vi "read_mote.vi"() -> (0 "DataSocket error":errorcluster, 1 "SF error":errorcluster)   [LabVIEW 2011]
panel:
  out "Sent Data":string
  out "Parsed Data":T1
  out "# Sent Data":u64
  out "Received data from mote":string
  out "Deque error":errorcluster
  # "DO NOT USE id 0 for a mote !"
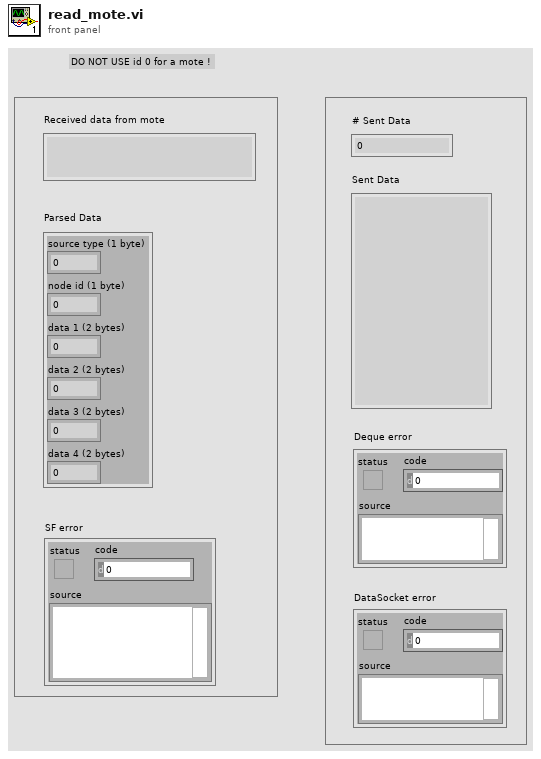
[diagram p1: front panel]
types:
  T1 = cluster{"source type (1 byte)":u8, "node id (1 byte)":u8, "data 1 (2 bytes)":u16, "data 2 (2 bytes)":u16, "data 3 (2 bytes)":u16, "data 4 (2 bytes)":u16}
  T2 = enum16{"Read", "Write", "ReadWrite", "BufferedRead", "BufferedReadWrite"}
  T3 = cluster{string, "data 1 (2 bytes)":u16, "data 2 (2 bytes)":u16, "data 3 (2 bytes)":u16, "data 4 (2 bytes)":u16, "date/time string":string, string, string}
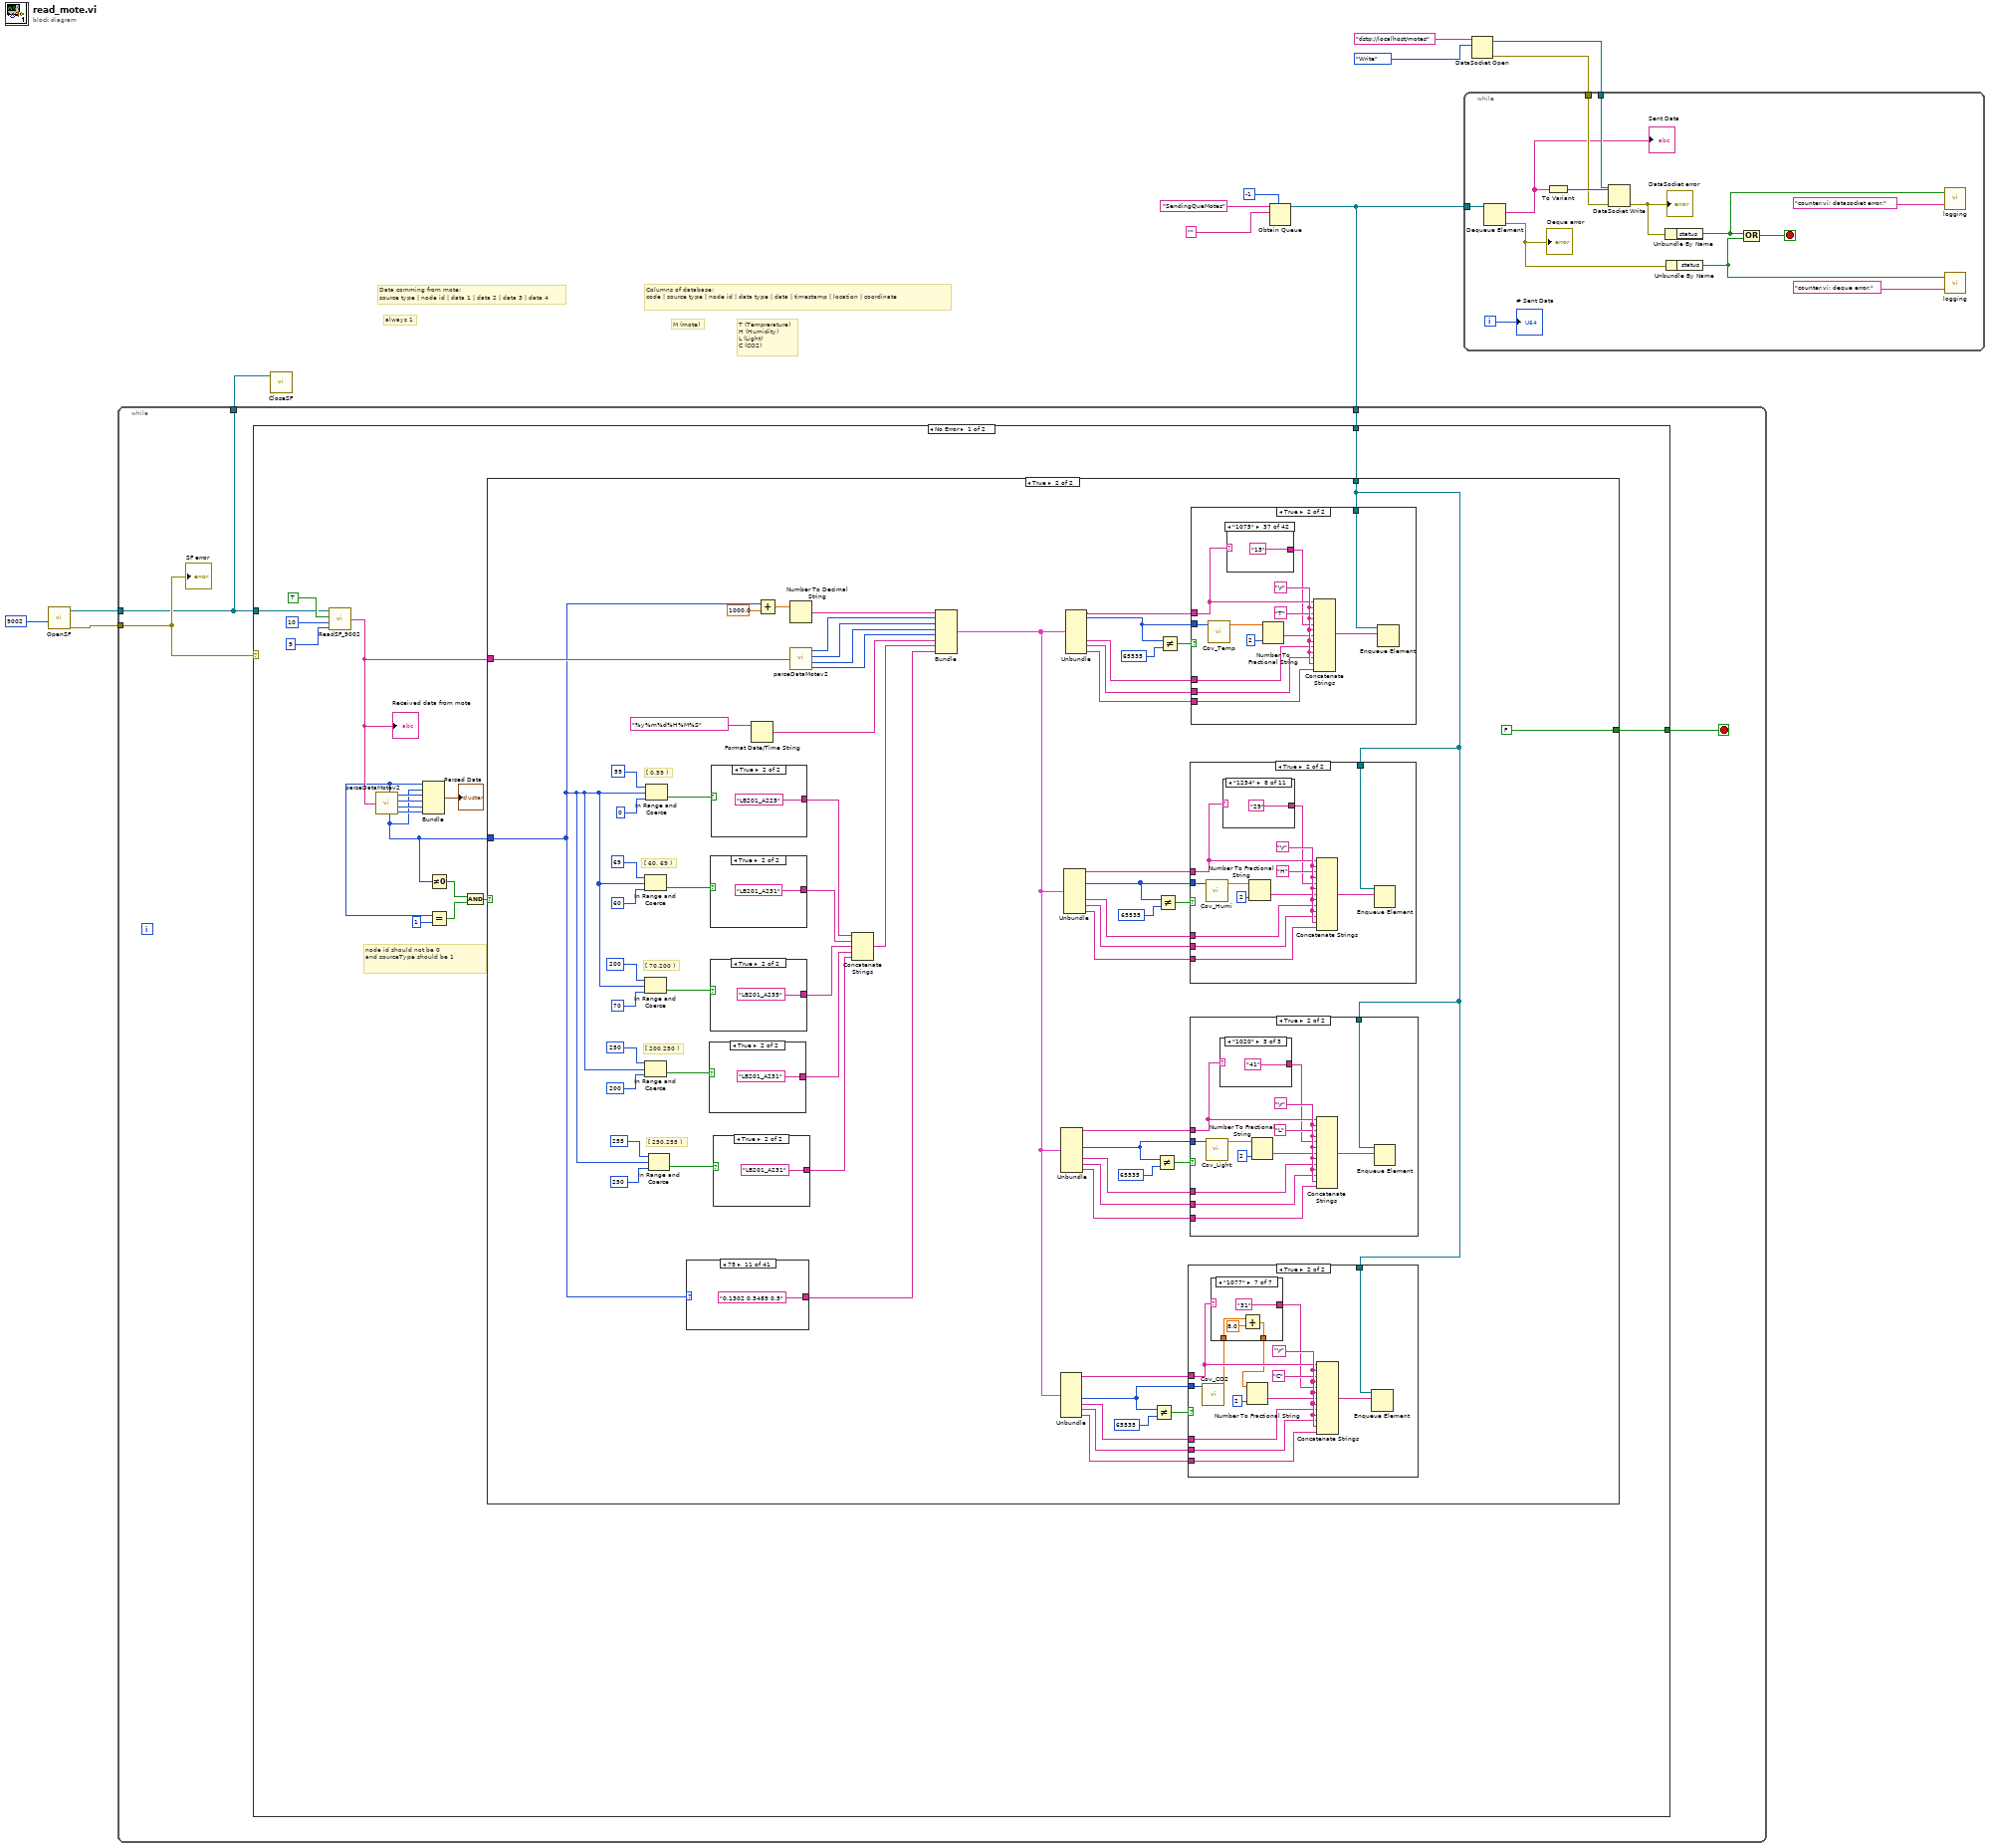
[diagram p0: block diagram]
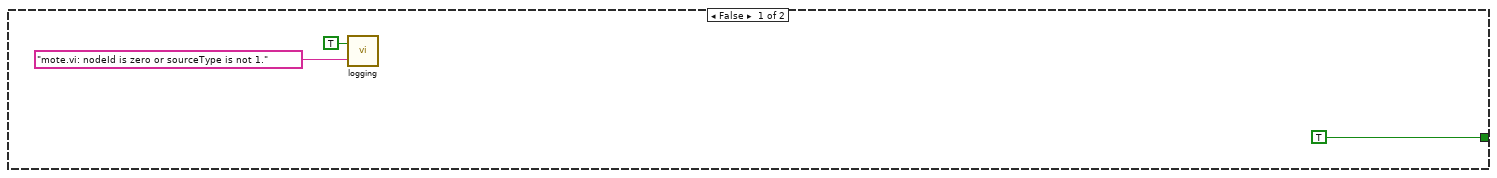
[diagram p2: hidden frame]
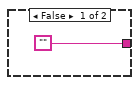
[diagram p3: hidden frame]
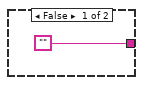
[diagram p4: hidden frame]
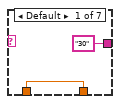
[diagram p6: hidden frame]
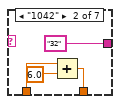
[diagram p7: hidden frame]
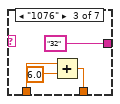
[diagram p8: hidden frame]
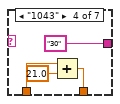
[diagram p9: hidden frame]
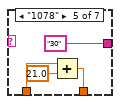
[diagram p10: hidden frame]
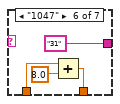
[diagram p11: hidden frame]
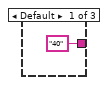
[diagram p13: hidden frame]
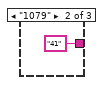
[diagram p14: hidden frame]
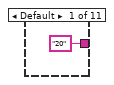
[diagram p16: hidden frame]
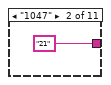
[diagram p17: hidden frame]
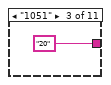
[diagram p18: hidden frame]
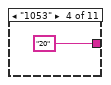
[diagram p19: hidden frame]
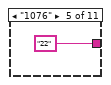
[diagram p20: hidden frame]
diagram:
  # "Data comming from mote:\nsource type | node id | data 1 | data 2 | data 3 | data 4"
  # "always 1"
  # "M (mote)"
  # "T (Temprerature)\nH (Humidity)\nL (Light)\nC (CO2)"
  # "Columns of database:\ncode | source type | node id | data type | data | timestamp | location | coordinate"
  n1 = call "OpenSF.vi"("port number"=u16 9002) -> ("error out"=w6:errorcluster, "connection ID"=w5:refnum<k5>)  [unwired: 1 out]
  n2 = Obtain Queue(max queue size (-1, unlimited)=-1, name (unnamed)="SendingQueMotes", element data type="") -> (queue out=w2:refnum<queue>)  [unwired: 2 in, 2 out]
  n3 = while {
    tunnel: w5 -> [w13]
    tunnel: w6 -> [w15]
    tunnel: w2 -> [w16]
    tunnel: [w13] -> w4
    stop <- w14 stop-if-true
    n4 = case shown="No Error" w15 {
      tunnel: w13 -> [w31 _]
      tunnel: w16 -> [w17 _]
      tunnel: [w30 TRUE] -> w14
      frame No Error {
        # "node id should not be 0\nand sourceType should be 1"
        n5 = call "ReadSF_9002.vi"("connection ID in"=w31, "enabled"=TRUE, "bytes to read"=10 ("f"), "header size"=9 ("bytes to read")) -> ("string"=w25:string)  [unwired: 2 in, 2 out]
        "Received data from mote" <- w25
        n6 = call "parseDataMotev2.vi"("input data"=w25) -> ("source type (1 byte)"=w22:u8, "node id (1 byte)"=w23:u8, "data 1 (2 bytes)"=w29:u16, "data 2 (2 bytes)"=w28:u16, "data 3 (2 bytes)"=w27:u16, "data 4 (2 bytes)"=w26:u16)
        n7 = Bundle("source type (1 byte)"=w22, "node id (1 byte)"=w23, "data 1 (2 bytes)"=w29, "data 2 (2 bytes)"=w28, "data 3 (2 bytes)"=w27, "data 4 (2 bytes)"=w26) -> (→"Parsed Data":T1)  [unwired: 1 in]
        n8 = Not Equal To 0?(x=w23) -> (x != 0?=w20:bool)
        n9 = Equal?(x=w22, y=u8 1) -> (x = y?=w19:bool)
        n10 = And(x=w20, y=w19) -> (x .and. y?=w18:bool)
        n11 = case shown="True" w18 {
          tunnel: w17 -> [_ w47]
          tunnel: w23 -> [_ w38]
          tunnel: [TRUE FALSE] -> w30
          tunnel: w25 -> [_ w86]
          frame False {
            n12 = call "logging.vi"("data"="mote.vi: nodeId is zero or sourceType is not 1.", "Boolean"=TRUE ("Enable")) -> ()  [unwired: 1 in]
          }
          frame True {
            # "[ 250,255 )"
            # "[ 60, 69 )"
            # "[ 200,250 )"
            # "[ 70,200 )"
            # "[ 0,59 )"
            n13 = In Range and Coerce(upper limit=u64 69, x=w38, lower limit=u64 60) -> (In Range?=w44:bool)  [unwired: 1 out]
            n14 = In Range and Coerce(upper limit=u64 200, x=w38, lower limit=u64 70) -> (In Range?=w93:bool)  [unwired: 1 out]
            n15 = In Range and Coerce(upper limit=u64 250, x=w38, lower limit=u64 200) -> (In Range?=w92:bool)  [unwired: 1 out]
            n16 = In Range and Coerce(upper limit=u64 59, x=w38, lower limit=u64 0) -> (In Range?=w94:bool)  [unwired: 1 out]
            n17 = In Range and Coerce(upper limit=u64 255, x=w38, lower limit=u64 250) -> (In Range?=w40:bool)  [unwired: 1 out]
            n18 = case shown="75" w38 {
              tunnel: ["0 0 0" "0.3711 0.3546 0.5" "0.3460 0.3361 0.5" "0.2781 0.0633 0.5" "0.2160 0.0575 0.5" "0.1595 0.4173 0.5" "0.0696 0.2006 0.5" "0.1152 0.3725 0.5" "0.0861 0.2026 0.5" "0.0081 0.2716 0.5" "0.1302 0.3489 0.5" "0.1693 0.4166 0.5" "0.1644 0.2875 0.5" "0.1024 0.3585 0.5" "0.1001 0.3125 0.5" "0.3226 0.3949 0.5" "0.3167 0.1137 0.5" "0.3885 0.0256 0.5" "0.3885 0.0256 0.5" "0.3243 0.0281 0.5" "0.3735 0.0300 0.5" "0.3000 0.0275 0.5" "0.3000 0.0275 0.5" "0.3000 0.0275 0.5" "0.3000 0.0275 0.5" "0.2874 0.2045 0.5" "0.3263 -0.0153 0.5" "0.3772 0.0377 0.5" "0.2953 0.0319 0.5" "0.3000 0.0319 0.5" "0.3019 0.0319 0.5" "0.3563 0.2090 0.5" "0.3046 0.3361 0.5" "0.3278 0.1419 0.5" "0.4208 0.2735 0.5" "0.2276 0.1834 0.5" "0.3383 0.3080 0.5" "0.3484 0.1987 0.5" "0.4062 0.1757 0.5" "0.3437 0.2076 0.5" "0.3118 0.3214 0.5"] -> w79
              frame Default {
              }
              frame 42 {
              }
              frame 2 {
              }
              frame 60 {
              }
              frame 61 {
              }
              frame 70 {
              }
              frame 71 {
              }
              frame 72 {
              }
              frame 73 {
              }
              frame 74 {
              }
              frame 75 {
              }
              frame 76 {
              }
              frame 77 {
              }
              frame 78 {
              }
              frame 79 {
              }
              frame 3 {
              }
              frame 47 {
              }
              frame 51 {
              }
              frame 55 {
              }
              frame 44 {
              }
              frame 46 {
              }
              frame 53 {
              }
              frame 52 {
              }
              frame 54 {
              }
              frame 45 {
              }
              frame 5 {
              }
              frame 6 {
              }
              frame 7 {
              }
              frame 8 {
              }
              frame 39 {
              }
              frame 9 {
              }
              frame 43 {
              }
              frame 11 {
              }
              frame 12 {
              }
              frame 110 {
              }
              frame 213 {
              }
              frame 20 {
              }
              frame 35 {
              }
              frame 36 {
              }
              frame 37 {
              }
              frame 33 {
              }
            }
            n19 = case shown="True" w92 {
              tunnel: ["" "LB201_A231"] -> w89
              frame False {
              }
              frame True {
              }
            }
            n20 = case shown="True" w44 {
              tunnel: ["" "LB201_A231"] -> w43
              frame False {
              }
              frame True {
              }
            }
            n21 = case shown="True" w93 {
              tunnel: ["" "LB201_A235"] -> w90
              frame False {
              }
              frame True {
              }
            }
            n22 = case shown="True" w94 {
              tunnel: ["" "LB201_A225"] -> w91
              frame False {
              }
              frame True {
              }
            }
            n23 = case shown="True" w40 {
              tunnel: ["" "LB201_A231"] -> w39
              frame False {
              }
              frame True {
              }
            }
            n24 = Format Date/Time String(time format string (%c)="%y%m%d%H%M%S") -> (date/time string=w81:string)  [unwired: 2 in]
            n25 = Add(x=w38, y=1000.0) -> (x+y=w49:dbl)
            n26 = Number To Decimal String(number=w49) -> (decimal integer string=w87:string)  [unwired: 1 in]
            n27 = call "parseDataMotev2.vi"("input data"=w86) -> ("data 1 (2 bytes)"=w85:u16, "data 2 (2 bytes)"=w84:u16, "data 3 (2 bytes)"=w83:u16, "data 4 (2 bytes)"=w82:u16)  [unwired: 2 out]
            n28 = Concatenate Strings(w91, w43, w90, w89, w39) -> (w80:string)
            n29 = Bundle(w87, "data 1 (2 bytes)"=w85, "data 2 (2 bytes)"=w84, "data 3 (2 bytes)"=w83, "data 4 (2 bytes)"=w82, "date/time string"=w81, w80, w79) -> (w78:T3)  [unwired: 1 in]
            n30 = Unbundle(w78) -> (w54:string, "data 4 (2 bytes)"=w53:u16, "date/time string"=w52:string, w51:string, w50:string)  [unwired: 3 out]
            n31 = Unbundle(w78) -> (w60:string, "data 3 (2 bytes)"=w55:u16, "date/time string"=w59:string, w58:string, w57:string)  [unwired: 3 out]
            n32 = Unbundle(w78) -> (w64:string, "data 2 (2 bytes)"=w56:u16, "date/time string"=w63:string, w62:string, w61:string)  [unwired: 3 out]
            n33 = Unbundle(w78) -> (w69:string, "data 1 (2 bytes)"=w68:u16, "date/time string"=w67:string, w66:string, w65:string)  [unwired: 3 out]
            n34 = Not Equal?(x=w53, y=u16 65535) -> (x != y?=w71:bool)
            n35 = Not Equal?(x=w55, y=u16 65535) -> (x != y?=w73:bool)
            n36 = Not Equal?(x=w56, y=u16 65535) -> (x != y?=w75:bool)
            n37 = Not Equal?(x=w68, y=u16 65535) -> (x != y?=w77:bool)
            n38 = case shown="True" w71 {
              tunnel: w53 -> [_ w119]
              tunnel: w52 -> [_ w113]
              tunnel: w47 -> [_ w118]
              tunnel: w54 -> [_ w110]
              tunnel: w51 -> [_ w112]
              tunnel: w50 -> [_ w111]
              frame False {
              }
              frame True {
                w115 = "\r"
                n39 = call "Cov_CO2.vi"("Input x"=w119) -> ("CO2"=w107:dbl)  [unwired: 10 in]
                n40 = case shown="\"1077\"" w110 {
                  tunnel: ["30" "32" "32" "30" "30" "31" "31"] -> w108
                  tunnel: w107 -> [w120 w124 w128 w132 w136 w139 w143]
                  tunnel: [w120 w122 w126 w130 w134 w138 w142] -> w106
                  frame Default {
                  }
                  frame "1042" {
                    n41 = Add(x=w124, y=6.0) -> (x+y=w122:dbl)
                  }
                  frame "1076" {
                    n42 = Add(x=w128, y=6.0) -> (x+y=w126:dbl)
                  }
                  frame "1043" {
                    n43 = Add(x=w132, y=21.0) -> (x+y=w130:dbl)
                  }
                  frame "1078" {
                    n44 = Add(x=w136, y=21.0) -> (x+y=w134:dbl)
                  }
                  frame "1047" {
                    n45 = Add(x=w139, y=8.0) -> (x+y=w138:dbl)
                  }
                  frame "1077" {
                    n46 = Add(x=w143, y=8.0) -> (x+y=w142:dbl)
                  }
                }
                n47 = Number To Fractional String(number=w106, precision (6)=i16 2) -> (F-format string=w114:string)  [unwired: 2 in]
                n48 = Concatenate Strings(w110, w115, "C", w115, w108, w115, w114, w115, w113, w115, w112, w115, w111) -> (w117:string)
                n49 = Enqueue Element(queue=w118, element=w117) -> ()  [unwired: 2 in, 3 out]
              }
            }
            n50 = case shown="True" w75 {
              tunnel: w64 -> [_ w164]
              tunnel: w56 -> [_ w174]
              tunnel: w47 -> [_ w173]
              tunnel: w63 -> [_ w167]
              tunnel: w62 -> [_ w166]
              tunnel: w61 -> [_ w165]
              frame False {
              }
              frame True {
                w169 = "\r"
                n51 = call "Cov_Humi.vi"("Input x"=w174) -> ("Humidity"=w171:dbl)  [unwired: 10 in]
                n52 = case shown="\"1254\"" w164 {
                  tunnel: ["20" "21" "20" "20" "22" "21" "20" "29" "23" "29" "22"] -> w162
                  frame Default {
                  }
                  frame "1047" {
                  }
                  frame "1051" {
                  }
                  frame "1053" {
                  }
                  frame "1076" {
                  }
                  frame "1077" {
                  }
                  frame "1078" {
                  }
                  frame "1254" {
                  }
                  frame "1012" {
                  }
                  frame "1006" {
                  }
                  frame "1042" {
                  }
                }
                n53 = Number To Fractional String(number=w171, precision (6)=i16 2) -> (F-format string=w168:string)  [unwired: 2 in]
                n54 = Concatenate Strings(w164, w169, "H", w169, w162, w169, w168, w169, w167, w169, w166, w169, w165) -> (w172:string)
                n55 = Enqueue Element(queue=w173, element=w172) -> ()  [unwired: 2 in, 3 out]
              }
            }
            n56 = case shown="True" w73 {
              tunnel: w60 -> [_ w148]
              tunnel: w55 -> [_ w157]
              tunnel: w59 -> [_ w151]
              tunnel: w47 -> [_ w158]
              tunnel: w58 -> [_ w150]
              tunnel: w57 -> [_ w149]
              frame False {
              }
              frame True {
                w153 = "\r"
                n57 = call "Cov_Light.vi"("Input x"=w157) -> ("Light"=w155:dbl)  [unwired: 10 in]
                n58 = case shown="\"1020\"" w148 {
                  tunnel: ["40" "41" "41"] -> w146
                  frame Default {
                  }
                  frame "1079" {
                  }
                  frame "1020" {
                  }
                }
                n59 = Number To Fractional String(number=w155, precision (6)=i16 2) -> (F-format string=w152:string)  [unwired: 2 in]
                n60 = Concatenate Strings(w148, w153, "L", w153, w146, w153, w152, w153, w151, w153, w150, w153, w149) -> (w156:string)
                n61 = Enqueue Element(queue=w158, element=w156) -> ()  [unwired: 2 in, 3 out]
              }
            }
            n62 = case shown="True" w77 {
              tunnel: w69 -> [_ w188]
              tunnel: w68 -> [_ w198]
              tunnel: w67 -> [_ w191]
              tunnel: w47 -> [_ w197]
              tunnel: w66 -> [_ w190]
              tunnel: w65 -> [_ w189]
              frame False {
              }
              frame True {
                w193 = "\r"
                n63 = call "Cov_Temp.vi"("Input x"=w198) -> ("Temperature"=w196:dbl)  [unwired: 10 in]
                n64 = case shown="\"1075\"" w188 {
                  tunnel: ["10" "11" "90" "90" "90" "90" "90" "15" "15" "1030" "1031" "1032" "16" "1034" "10" "15" "16" "1038" "17" "1040" "13" "15" "15" "91" "91" "91" "91" "92" "15" "15" "15" "16" "90" "16" "15" "15" "13" "12" "11" "10" "15" "12"] -> w186
                  frame Default {
                  }
                  frame "1047" {
                  }
                  frame "1051" {
                  }
                  frame "1053" {
                  }
                  frame "1054" {
                  }
                  frame "1045" {
                  }
                  frame "1052" {
                  }
                  frame "1110" {
                  }
                  frame "1006" {
                  }
                  frame "1030" {
                  }
                  frame "1031" {
                  }
                  frame "1032" {
                  }
                  frame "1033" {
                  }
                  frame "1034" {
                  }
                  frame "1035" {
                  }
                  frame "1036" {
                  }
                  frame "1037" {
                  }
                  frame "1038" {
                  }
                  frame "1039" {
                  }
                  frame "1040" {
                  }
                  frame "1012" {
                  }
                  frame "1005" {
                  }
                  frame "1007" {
                  }
                  frame "1008" {
                  }
                  frame "1044" {
                  }
                  frame "1046" {
                  }
                  frame "1055" {
                  }
                  frame "1009" {
                  }
                  frame "1151" {
                  }
                  frame "1060" {
                  }
                  frame "1061" {
                  }
                  frame "1070" {
                  }
                  frame "1071" {
                  }
                  frame "1072" {
                  }
                  frame "1073" {
                  }
                  frame "1074" {
                  }
                  frame "1075" {
                  }
                  frame "1076" {
                  }
                  frame "1077" {
                  }
                  frame "1078" {
                  }
                  frame "1011" {
                  }
                  frame "1042" {
                  }
                }
                n65 = Number To Fractional String(number=w196, precision (6)=i16 2) -> (F-format string=w192:string)  [unwired: 2 in]
                n66 = Concatenate Strings(w188, w193, "T", w193, w186, w193, w192, w193, w191, w193, w190, w193, w189) -> (w194:string)
                n67 = Enqueue Element(queue=w197, element=w194) -> ()  [unwired: 2 in, 3 out]
              }
            }
          }
        }
      }
      frame Error {
        n68 = call "logging.vi"("data"="mote.vi: Error in SF", "Boolean"=TRUE ("Enable")) -> ()  [unwired: 1 in]
      }
    }
    "SF error" <- w15
  }
  n69 = call "CloseSF.vi"("connection ID"=w4) -> ()  [unwired: 2 in]
  n70 = DataSocket Open(10:T2."Write" ("mode"), 11:"dstp://localhost/motes" ("URL 3")) -> (0:w7:errorcluster, 3:w8:refnum<k13>)  [unwired: 2 in]
  n71 = while {
    tunnel: w2 -> [w303]
    tunnel: w8 -> [w302]
    tunnel: w7 -> [w298]
    i -> [w297]
    stop <- w292 stop-if-true
    n72 = Dequeue Element(queue=w303) -> (element=w291:string, error out=w300:errorcluster)  [unwired: 2 in, 2 out]
    "Deque error" <- w300
    "Sent Data" <- w291
    n73 = To Variant(anything=w291) -> (Variant=w301:variant)
    n74 = DataSocket Write(8:w298, 10:w301, 11:w302) -> (0:w299:errorcluster)  [unwired: 3 out]
    "DataSocket error" <- w299
    n75 = Unbundle By Name(w299) -> ("status"=w294:bool)
    n76 = Unbundle By Name(w300) -> ("status"=w293:bool)
    n77 = Compound Arithmetic op=OR(w294, w293) -> (w292:bool)
    n78 = call "logging.vi"("data"="counter.vi: datasocket error.", "Boolean"=w294) -> ()  [unwired: 1 in]
    n79 = call "logging.vi"("data"="counter.vi: deque error.", "Boolean"=w293) -> ()  [unwired: 1 in]
    "# Sent Data" <- w297
  }
